vi "unn.vi"(0 "Array":u32[][](array[numeric]), 3 "cx":u16, 7 "cy":u16) -> (20 "u02":T1, 21 "u03":T1, 22 "u11":T1, 23 "u12":T1, 24 "u20":T1, 25 "u21":T1, 26 "u30":T1)   [LabVIEW 2021]
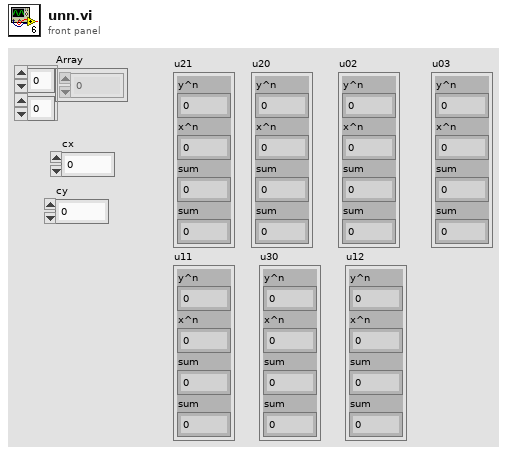
[diagram p1: front panel]
types:
  T1 = cluster{"y^n":dbl, "x^n":dbl, "sum":dbl, "sum":dbl}
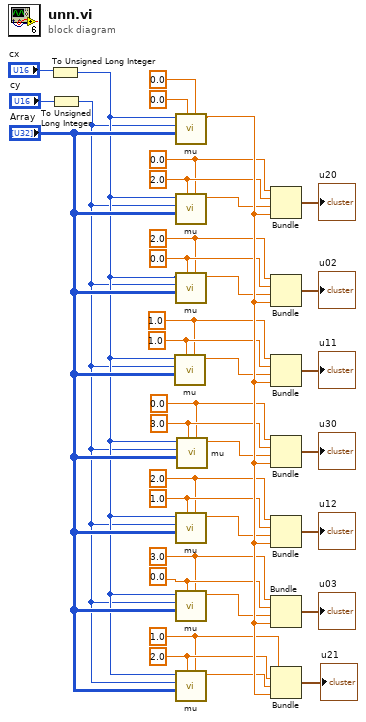
[diagram p0: block diagram]
diagram:
  w24 = 1.0 ("y^n")
  w25 = 2.0 ("x^n")
  w21 = 3.0 ("y^n")
  w22 = 0.0 ("x^n")
  w19 = 2.0 ("y^n")
  w20 = 1.0 ("x^n")
  w17 = 0.0 ("y^n")
  w18 = 3.0 ("x^n")
  w11 = 0.0 ("y^n")
  w12 = 2.0 ("x^n")
  w13 = 2.0 ("y^n")
  w14 = 0.0 ("x^n")
  w15 = 1.0 ("y^n")
  w16 = 1.0 ("x^n")
  n1 = To Unsigned Long Integer(number="cx") -> (unsigned 32bit integer=w3:u32)
  n2 = To Unsigned Long Integer(number="cy") -> (unsigned 32bit integer=w1:u32)
  n3 = call "mu.vi"("q"=w15, "p"=w16, "Array"="Array", "cy"=w1, "cx"=w3) -> ("sum"=w30:dbl)  [unwired: 6 in]
  n4 = call "mu.vi"("q"=0.0 ("y^n"), "p"=0.0 ("x^n"), "Array"="Array", "cy"=w1, "cx"=w3) -> ("sum"=w33:dbl)  [unwired: 6 in]
  n5 = call "mu.vi"("q"=w11, "p"=w12, "Array"="Array", "cy"=w1, "cx"=w3) -> ("sum"=w32:dbl)  [unwired: 6 in]
  n6 = call "mu.vi"("q"=w13, "p"=w14, "Array"="Array", "cy"=w1, "cx"=w3) -> ("sum"=w31:dbl)  [unwired: 6 in]
  n7 = call "mu.vi"("q"=w19, "p"=w20, "Array"="Array", "cy"=w1, "cx"=w3) -> ("sum"=w28:dbl)  [unwired: 6 in]
  n8 = call "mu.vi"("q"=w21, "p"=w22, "Array"="Array", "cy"=w1, "cx"=w3) -> ("sum"=w27:dbl)  [unwired: 6 in]
  n9 = call "mu.vi"("q"=w24, "p"=w25, "Array"="Array", "cy"=w1, "cx"=w3) -> ("sum"=w26:dbl)  [unwired: 6 in]
  n10 = call "mu.vi"("q"=w17, "p"=w18, "Array"="Array", "cy"=w1, "cx"=w3) -> ("sum"=w29:dbl)  [unwired: 6 in]
  n11 = Bundle("y^n"=w11, "x^n"=w12, "sum"=w32, "sum"=w33) -> (→"u20":T1)  [unwired: 1 in]
  n12 = Bundle("y^n"=w13, "x^n"=w14, "sum"=w31, "sum"=w33) -> (→"u02":T1)  [unwired: 1 in]
  n13 = Bundle("y^n"=w15, "x^n"=w16, "sum"=w30, "sum"=w33) -> (→"u11":T1)  [unwired: 1 in]
  n14 = Bundle("y^n"=w17, "x^n"=w18, "sum"=w29, "sum"=w33) -> (→"u30":T1)  [unwired: 1 in]
  n15 = Bundle("y^n"=w19, "x^n"=w20, "sum"=w28, "sum"=w33) -> (→"u12":T1)  [unwired: 1 in]
  n16 = Bundle("y^n"=w21, "x^n"=w22, "sum"=w27, "sum"=w33) -> (→"u03":T1)  [unwired: 1 in]
  n17 = Bundle("y^n"=w24, "x^n"=w25, "sum"=w26, "sum"=w33) -> (→"u21":T1)  [unwired: 1 in]
